vi "GeoData.vi"() -> ()   [LabVIEW 2017] (continued)
41013\tPost\tOR\tCrook County\tH1\n97756\t41013\tRedmond\tOR\tCrook County\tH1\n97406\t41015\tAgness\tOR\tCurry County\tH1\n97450\t41015\tLanglois\tOR\tCurry County\tH1\n97491\t41015\tWedderburn\tOR\tCurry County\tH1\n97444\t41015\tGold beach\tOR\tCurry County\tH1\n97476\t41015\tSixes\tOR\tCurry County\tH1\n97415\t41015\tBrookings\tOR\tCurry County\tH1\n97465\t41015\tPort orford\tOR\tCurry County\tH1\n97464\t41015\tOphir\tOR\tCurry County\tH1\n97709\t41017\tBend\tOR\tDeschutes County\tH1\n97701\t41017\tBend\tOR\tDeschutes County\tH1\n97759\t41017\tSisters\tOR\tDeschutes County\tH1\n97760\t41017\tTerrebonne\tOR\tDeschutes County\tH1\n97708\t41017\tBend\tOR\tDeschutes County\tH1\n97702\t41017\tBend\tOR\tDeschutes County\tH1\n97703\t41017\tBend\tOR\tDeschutes County\tH1\n97739\t41017\tLa pine\tOR\tDeschutes County\tH1\n97756\t41017\tRedmond\tOR\tDeschutes County\tH1\n97707\t41017\tBend\tOR\tDeschutes County\tH1\n97712\t41017\tBrothers\tOR\tDeschutes County\tH1\n97473\t41019\tScottsburg\tOR\tDouglas County\tH1\n97471\t41019\tRoseburg\tOR\tDouglas County\tH1\n97432\t41019\tDillard\tOR\tDouglas County\tH1\n97410\t41019\tAzalea\tOR\tDouglas County\tH1\n97443\t41019\tGlide\tOR\tDouglas County\tH1\n97481\t41019\tTenmile\tOR\tDouglas County\tH1\n97429\t41019\tDays creek\tOR\tDouglas County\tH1\n97442\t41019\tGlendale\tOR\tDouglas County\tH1\n97417\t41019\tCanyonville\tOR\tDouglas County\tH1\n97459\t41019\tNorth bend\tOR\tDouglas County\tH1\n97470\t41019\tRoseburg\tOR\tDouglas County\tH1\n97462\t41019\tOakland\tOR\tDouglas County\tH1\n97467\t41019\tReedsport\tOR\tDouglas County\tH1\n97469\t41019\tRiddle\tOR\tDouglas County\tH1\n97496\t41019\tWinston\tOR\tDouglas County\tH1\n97731\t41019\tChemult\tOR\tDouglas County\tH1\n97424\t41019\tCottage grove\tOR\tDouglas County\tH1\n97499\t41019\tYoncalla\tOR\tDouglas County\tH1\n97436\t41019\tElkton\tOR\tDouglas County\tH1\n97495\t41019\tWinchester\tOR\tDouglas County\tH1\n97486\t41019\tUmpqua\tOR\tDouglas County\tH1\n97441\t41019\tGardiner\tOR\tDouglas County\tH1\n97457\t41019\tMyrtle creek\tOR\tDouglas County\tH1\n97447\t41019\tIdleyld park\tOR\tDouglas County\tH1\n97435\t41019\tDrain\tOR\tDouglas County\tH1\n97493\t41019\tWestlake\tOR\tDouglas County\tH1\n97484\t41019\tTiller\tOR\tDouglas County\tH1\n97479\t41019\tSutherlin\tOR\tDouglas County\tH1\n97416\t41019\tCamas valley\tOR\tDouglas County\tH1\n97494\t41019\tWilbur\tOR\tDouglas County\tH1\n97843\t41021\tIone\tOR\tGilliam County\tH1\n97812\t41021\tArlington\tOR\tGilliam County\tH1\n97830\t41021\tFossil\tOR\tGilliam County\tH1\n97823\t41021\tCondon\tOR\tGilliam County\tH1\n97865\t41023\tMount vernon\tOR\tGrant County\tH1\n97856\t41023\tLong creek\tOR\tGrant County\tH1\n97820\t41023\tCanyon city\tOR\tGrant County\tH1\n97864\t41023\tMonument\tOR\tGrant County\tH1\n97817\t41023\tBates\tOR\tGrant County\tH1\n97825\t41023\tDayville\tOR\tGrant County\tH1\n97848\t41023\tKimberly\tOR\tGrant County\tH1\n97877\t41023\tSumpter\tOR\tGrant County\tH1\n97845\t41023\tJohn day\tOR\tGrant County\tH1\n97869\t41023\tPrairie city\tOR\tGrant County\tH1\n97873\t41023\tSeneca\tOR\tGrant County\tH1\n97710\t41025\tFields\tOR\tHarney County\tH1\n97721\t41025\tPrinceton\tOR\tHarney County\tH1\n97736\t41025\tFrenchglen\tOR\tHarney County\tH1\n97732\t41025\tCrane\tOR\tHarney County\tH1\n97758\t41025\tRiley\tOR\tHarney County\tH1\n97720\t41025\tBurns\tOR\tHarney County\tH1\n97904\t41025\tDrewsey\tOR\tHarney County\tH1\n97738\t41025\tHines\tOR\tHarney County\tH1\n97722\t41025\tDiamond\tOR\tHarney County\tH1\n97044\t41027\tOdell\tOR\tHood River County\tH1\n97014\t41027\tCascade locks\tOR\tHood River County\tH1\n97031\t41027\tHood river\tOR\tHood River County\tH1\n97041\t41027\tMount hood parkdale\tOR\tHood River County\tH1\n97526\t41029\tGrants pass\tOR\tJackson County\tH1\n97541\t41029\tTrail\tOR\tJackson County\tH1\n97502\t41029\tCentral point\tOR\tJackson County\tH1\n97524\t41029\tEagle point\tOR\tJackson County\tH1\n97527\t41029\tGrants pass\tOR\tJackson County\tH1\n97504\t41029\tMedford\tOR\tJackson County\tH1\n97530\t41029\tJacksonville\tOR\tJackson County\tH1\n97537\t41029\tRogue river\tOR\tJackson County\tH1\n97539\t41029\tShady cove\tOR\tJackson County\tH1\n97535\t41029\tPhoenix\tOR\tJackson County\tH1\n97520\t41029\tAshland\tOR\tJackson County\tH1\n97497\t41029\tWolf creek\tOR\tJackson County\tH1\n97540\t41029\tTalent\tOR\tJackson County\tH1\n97544\t41029\tWilliams\tOR\tJackson County\tH1\n97501\t41029\tMedford\tOR\tJackson County\tH1\n97503\t41029\tWhite city\tOR\tJackson County\tH1\n97525\t41029\tGold hill\tOR\tJackson County\tH1\n97522\t41029\tButte falls\tOR\tJackson County\tH1\n97536\t41029\tProspect\tOR\tJackson County\tH1\n97761\t41031\tWarm springs\tOR\tJefferson County\tH1\n97759\t41031\tSisters\tOR\tJefferson County\tH1\n97741\t41031\tMadras\tOR\tJefferson County\tH1\n97760\t41031\tTerrebonne\tOR\tJefferson County\tH1\n97711\t41031\tAshwood\tOR\tJefferson County\tH1\n97734\t41031\tCulver\tOR\tJefferson County\tH1\n97730\t41031\tCamp sherman\tOR\tJefferson County\tH1\n97526\t41033\tGrants pass\tOR\tJosephine County\tH1\n97531\t41033\tKerby\tOR\tJosephine County\tH1\n97527\t41033\tGrants pass\tOR\tJosephine County\tH1\n97543\t41033\tWilderville\tOR\tJosephine County\tH1\n97528\t41033\tGrants pass\tOR\tJosephine County\tH1\n97530\t41033\tJacksonville\tOR\tJosephine County\tH1\n97523\t41033\tCave junction\tOR\tJosephine County\tH1\n97532\t41033\tMerlin\tOR\tJosephine County\tH1\n97497\t41033\tWolf creek\tOR\tJosephine County\tH1\n97534\t41033\tO brien\tOR\tJosephine County\tH1\n97533\t41033\tMurphy\tOR\tJosephine County\tH1\n97544\t41033\tWilliams\tOR\tJosephine County\tH1\n97538\t41033\tSelma\tOR\tJosephine County\tH1\n97603\t41035\tKlamath falls\tOR\tKlamath County\tH1\n97601\t41035\tKlamath falls\tOR\tKlamath County\tH1\n97623\t41035\tBonanza\tOR\tKlamath County\tH1\n97627\t41035\tKeno\tOR\tKlamath County\tH1\n97621\t41035\tBeatty\tOR\tKlamath County\tH1\n97602\t41035\tKlamath falls\tOR\tKlamath County\tH1\n97604\t41035\tCrater lake\tOR\tKlamath County\tH1\n97625\t41035\tDairy\tOR\tKlamath County\tH1\n97731\t41035\tChemult\tOR\tKlamath County\tH1\n97739\t41035\tLa pine\tOR\tKlamath County\tH1\n97634\t41035\tMidland\tOR\tKlamath County\tH1\n97622\t41035\tBly\tOR\tKlamath County\tH1\n97624\t41035\tChiloquin\tOR\tKlamath County\tH1\n97733\t41035\tCrescent\tOR\tKlamath County\tH1\n97632\t41035\tMalin\tOR\tKlamath County\tH1\n97639\t41035\tSprague river\tOR\tKlamath County\tH1\n97626\t41035\tFort klamath\tOR\tKlamath County\tH1\n97633\t41035\tMerrill\tOR\tKlamath County\tH1\n97737\t41035\tGilchrist\tOR\tKlamath County\tH1\n97640\t41037\tSummer lake\tOR\tLake County\tH1\n97637\t41037\tPlush\tOR\tLake County\tH1\n97630\t41037\tLakeview\tOR\tLake County\tH1\n97641\t41037\tChristmas valley\tOR\tLake County\tH1\n97620\t41037\tAdel\tOR\tLake County\tH1\n97635\t41037\tNew pine creek\tOR\tLake County\tH1\n97638\t41037\tSilver lake\tOR\tLake County\tH1\n97735\t41037\tFort rock\tOR\tLake County\tH1\n97636\t41037\tPaisley\tOR\tLake County\tH1\n97413\t41039\tBlue river\tOR\tLane County\tH1\n97412\t41039\tBlachly\tOR\tLane County\tH1\n97402\t41039\tEugene\tOR\tLane County\tH1\n97404\t41039\tEugene\tOR\tLane County\tH1\n97454\t41039\tMarcola\tOR\tLane County\tH1\n97426\t41039\tCreswell\tOR\tLane County\tH1\n97487\t41039\tVeneta\tOR\tLane County\tH1\n97451\t41039\tLorane\tOR\tLane County\tH1\n97498\t41039\tYachats\tOR\tLane County\tH1\n97488\t41039\tVida\tOR\tLane County\tH1\n97461\t41039\tNoti\tOR\tLane County\tH1\n97324\t41039\tAlsea\tOR\tLane County\tH1\n97401\t41039\tEugene\tOR\tLane County\tH1\n97477\t41039\tSpringfield\tOR\tLane County\tH1\n97478\t41039\tSpringfield\tOR\tLane County\tH1\n97434\t41039\tDorena\tOR\tLane County\tH1\n97446\t41039\tHarrisburg\tOR\tLane County\tH1\n97463\t41039\tOakridge\tOR\tLane County\tH1\n97492\t41039\tWestfir\tOR\tLane County\tH1\n97409\t41039\tAlvadore\tOR\tLane County\tH1\n97438\t41039\tFall creek\tOR\tLane County\tH1\n97390\t41039\tTidewater\tOR\tLane County\tH1\n97490\t41039\tWalton\tOR\tLane County\tH1\n97489\t41039\tWalterville\tOR\tLane County\tH1\n97448\t41039\tJunction city\tOR\tLane County\tH1\n97453\t41039\tMapleton\tOR\tLane County\tH1\n97456\t41039\tMonroe\tOR\tLane County\tH1\n97480\t41039\tSwisshome\tOR\tLane County\tH1\n97405\t41039\tEugene\tOR\tLane County\tH1\n97424\t41039\tCottage grove\tOR\tLane County\tH1\n97439\t41039\tFlorence\tOR\tLane County\tH1\n97419\t41039\tCheshire\tOR\tLane County\tH1\n97437\t41039\tElmira\tOR\tLane County\tH1\n97452\t41039\tLowell\tOR\tLane County\tH1\n97430\t41039\tDeadwood\tOR\tLane County\tH1\n97408\t41039\tEugene\tOR\tLane County\tH1\n97493\t41039\tWestlake\tOR\tLane County\tH1\n97403\t41039\tEugene\tOR\tLane County\tH1\n97440\t41039\tEugene\tOR\tLane County\tH1\n97455\t41039\tPleasant hill\tOR\tLane County\tH1\n97475\t41039\tSpringfield\tOR\tLane County\tH1\n97431\t41039\tDexter\tOR\tLane County\tH1\n97394\t41041\tWaldport\tOR\tLincoln County\tH1\n97498\t41041\tYachats\tOR\tLincoln County\tH1\n97369\t41041\tOtter rock\tOR\tLincoln County\tH1\n97324\t41041\tAlsea\tOR\tLincoln County\tH1\n97391\t41041\tToledo\tOR\tLincoln County\tH1\n97364\t41041\tNeotsu\tOR\tLincoln County\tH1\n97367\t41041\tLincoln city\tOR\tLincoln County\tH1\n97390\t41041\tTidewater\tOR\tLincoln County\tH1\n97341\t41041\tDepoe bay\tOR\tLincoln County\tH1\n97380\t41041\tSiletz\tOR\tLincoln County\tH1\n97343\t41041\tEddyville\tOR\tLincoln County\tH1\n97388\t41041\tGleneden beach\tOR\tLincoln County\tH1\n97357\t41041\tLogsden\tOR\tLincoln County\tH1\n97376\t41041\tSeal rock\tOR\tLincoln County\tH1\n97365\t41041\tNewport\tOR\tLincoln County\tH1\n97368\t41041\tOtis\tOR\tLincoln County\tH1\n97366\t41041\tSouth beach\tOR\tLincoln County\tH1\n97326\t41041\tBlodgett\tOR\tLincoln County\tH1\n97346\t41043\tGates\tOR\tLinn County\tH1\n97333\t41043\tCorvallis\tOR\tLinn County\tH1\n97374\t41043\tScio\tOR\tLinn County\tH1\n97446\t41043\tHarrisburg\tOR\tLinn County\tH1\n97336\t41043\tCrawfordsville\tOR\tLinn County\tH1\n97355\t41043\tLebanon\tOR\tLinn County\tH1\n97383\t41043\tStayton\tOR\tLinn County\tH1\n97386\t41043\tSweet home\tOR\tLinn County\tH1\n97360\t41043\tMill city\tOR\tLinn County\tH1\n97350\t41043\tIdanha\tOR\tLinn County\tH1\n97327\t41043\tBrownsville\tOR\tLinn County\tH1\n97389\t41043\tTangent\tOR\tLinn County\tH1\n97377\t41043\tShedd\tOR\tLinn County\tH1\n97329\t41043\tCascadia\tOR\tLinn County\tH1\n97348\t41043\tHalsey\tOR\tLinn County\tH1\n97335\t41043\tCrabtree\tOR\tLinn County\tH1\n97358\t41043\tLyons\tOR\tLinn County\tH1\n97345\t41043\tFoster\tOR\tLinn County\tH1\n97322\t41043\tAlbany\tOR\tLinn County\tH1\n97321\t41043\tAlbany\tOR\tLinn County\tH1\n97352\t41043\tJefferson\tOR\tLinn County\tH1\n97906\t41045\tHarper\tOR\tMalheur County\tH1\n97908\t41045\tIronside\tOR\tMalheur County\tH1\n97910\t41045\tJordan valley\tOR\tMalheur County\tH1\n97920\t41045\tWestfall\tOR\tMalheur County\tH1\n97903\t41045\tBrogan\tOR\tMalheur County\tH1\n97918\t41045\tVale\tOR\tMalheur County\tH1\n97911\t41045\tJuntura\tOR\tMalheur County\tH1\n97913\t41045\tNyssa\tOR\tMalheur County\tH1\n97917\t41045\tRiverside\tOR\tMalheur County\tH1\n97902\t41045\tArock\tOR\tMalheur County\tH1\n97901\t41045\tAdrian\tOR\tMalheur County\tH1\n97909\t41045\tJamieson\tOR\tMalheur County\tH1\n97914\t41045\tOntario\tOR\tMalheur County\tH1\n97907\t41045\tHuntington\tOR\tMalheur County\tH1\n97137\t41047\tSaint paul\tOR\tMarion County\tH1\n97301\t41047\tSalem\tOR\tMarion County\tH1\n97346\t41047\tGates\tOR\tMarion County\tH1\n97342\t41047\tDetroit\tOR\tMarion County\tH1\n97306\t41047\tSalem\tOR\tMarion County\tH1\n97362\t41047\tMount angel\tOR\tMarion County\tH1\n97026\t41047\tGervais\tOR\tMarion County\tH1\n97308\t41047\tSalem\tOR\tMarion County\tH1\n97310\t41047\tSalem\tOR\tMarion County\tH1\n97373\t41047\tSaint benedict\tOR\tMarion County\tH1\n97317\t41047\tSalem\tOR\tMarion County\tH1\n97381\t41047\tSilverton\tOR\tMarion County\tH1\n97385\t41047\tSublimity\tOR\tMarion County\tH1\n97375\t41047\tScotts mills\tOR\tMarion County\tH1\n97071\t41047\tWoodburn\tOR\tMarion County\tH1\n97307\t41047\tKeizer\tOR\tMarion County\tH1\n97392\t41047\tTurner\tOR\tMarion County\tH1\n97383\t41047\tStayton\tOR\tMarion County\tH1\n97384\t41047\tMehama\tOR\tMarion County\tH1\n97360\t41047\tMill city\tOR\tMarion County\tH1\n97350\t41047\tIdanha\tOR\tMarion County\tH1\n97314\t41047\tSalem\tOR\tMarion County\tH1\n97358\t41047\tLyons\tOR\tMarion County\tH1\n97311\t41047\tSalem\tOR\tMarion County\tH1\n97312\t41047\tSalem\tOR\tMarion County\tH1\n97002\t41047\tAurora\tOR\tMarion County\tH1\n97302\t41047\tSalem\tOR\tMarion County\tH1\n97303\t41047\tSalem\tOR\tMarion County\tH1\n97020\t41047\tDonald\tOR\tMarion County\tH1\n97309\t41047\tSalem\tOR\tMarion County\tH1\n97325\t41047\tAumsville\tOR\tMarion County\tH1\n97305\t41047\tSalem\tOR\tMarion County\tH1\n97032\t41047\tHubbard\tOR\tMarion County\tH1\n97352\t41047\tJefferson\tOR\tMarion County\tH1\n97313\t41047\tSalem\tOR\tMarion County\tH1\n97843\t41049\tIone\tOR\tMorrow County\tH1\n97839\t41049\tLexington\tOR\tMorrow County\tH1\n97826\t41049\tEcho\tOR\tMorrow County\tH1\n97818\t41049\tBoardman\tOR\tMorrow County\tH1\n97836\t41049\tHeppner\tOR\tMorrow County\tH1\n97823\t41049\tCondon\tOR\tMorrow County\tH1\n97844\t41049\tIrrigon\tOR\tMorrow County\tH1\n97838\t41049\tHermiston\tOR\tMorrow County\tH1\n97882\t41049\tUmatilla\tOR\tMorrow County\tH1\n97205\t41051\tPortland\tOR\tMultnomah County\tH1\n97209\t41051\tPortland\tOR\tMultnomah County\tH1\n97221\t41051\tPortland\tOR\tMultnomah County\tH1\n97215\t41051\tPortland\tOR\tMultnomah County\tH1\n97286\t41051\tPortland\tOR\tMultnomah County\tH1\n97292\t41051\tPortland\tOR\tMultnomah County\tH1\n97293\t41051\tPortland\tOR\tMultnomah County\tH1\n97283\t41051\tPortland\tOR\tMultnomah County\tH1\n97253\t41051\tPortland\tOR\tMultnomah County\tH1\n97133\t41051\tNorth plains\tOR\tMultnomah County\tH1\n97220\t41051\tPortland\tOR\tMultnomah County\tH1\n97216\t41051\tPortland\tOR\tMultnomah County\tH1\n97217\t41051\tPortland\tOR\tMultnomah County\tH1\n97009\t41051\tBoring\tOR\tMultnomah County\tH1\n97208\t41051\tPortland\tOR\tMultnomah County\tH1\n97254\t41051\tPortland\tOR\tMultnomah County\tH1\n97206\t41051\tPortland\tOR\tMultnomah County\tH1\n97233\t41051\tPortland\tOR\tMultnomah County\tH1\n97296\t41051\tPortland\tOR\tMultnomah County\tH1\n97207\t41051\tPortland\tOR\tMultnomah County\tH1\n97203\t41051\tPortland\tOR\tMultnomah County\tH1\n97210\t41051\tPortland\tOR\tMultnomah County\tH1\n97236\t41051\tPortland\tOR\tMultnomah County\tH1\n97266\t41051\tPortland\tOR\tMultnomah County\tH1\n97204\t41051\tPortland\tOR\tMultnomah County\tH1\n97223\t41051\tPortland\tOR\tMultnomah County\tH1\n97225\t41051\tPortland\tOR\tMultnomah County\tH1\n97227\t41051\tPortland\tOR\tMultnomah County\tH1\n97218\t41051\tPortland\tOR\tMultnomah County\tH1\n97231\t41051\tPortland\tOR\tMultnomah County\tH1\n97030\t41051\tGresham\tOR\tMultnomah County\tH1\n97014\t41051\tCascade locks\tOR\tMultnomah County\tH1\n97060\t41051\tTroutdale\tOR\tMultnomah County\tH1\n97019\t41051\tCorbett\tOR\tMultnomah County\tH1\n97294\t41051\tPortland\tOR\tMultnomah County\tH1\n97238\t41051\tPortland\tOR\tMultnomah County\tH1\n97280\t41051\tPortland\tOR\tMultnomah County\tH1\n97290\t41051\tPortland\tOR\tMultnomah County\tH1\n97242\t41051\tPortland\tOR\tMultnomah County\tH1\n97282\t41051\tPortland\tOR\tMultnomah County\tH1\n97250\t41051\tPortland\tOR\tMultnomah County\tH1\n97214\t41051\tPortland\tOR\tMultnomah County\tH1\n97219\t41051\tPortland\tOR\tMultnomah County\tH1\n97024\t41051\tFairview\tOR\tMultnomah County\tH1\n97056\t41051\tScappoose\tOR\tMultnomah County\tH1\n97251\t41051\tPortland\tOR\tMultnomah County\tH1\n97201\t41051\tPortland\tOR\tMultnomah County\tH1\n97124\t41051\tHillsboro\tOR\tMultnomah County\tH1\n97211\t41051\tPortland\tOR\tMultnomah County\tH1\n97212\t41051\tPortland\tOR\tMultnomah County\tH1\n97222\t41051\tPortland\tOR\tMultnomah County\tH1\n97229\t41051\tPortland\tOR\tMultnomah County\tH1\n97239\t41051\tPortland\tOR\tMultnomah County\tH1\n97080\t41051\tGresham\tOR\tMultnomah County\tH1\n97202\t41051\tPortland\tOR\tMultnomah County\tH1\n97213\t41051\tPortland\tOR\tMultnomah County\tH1\n97230\t41051\tPortland\tOR\tMultnomah County\tH1\n97232\t41051\tPortland\tOR\tMultnomah County\tH1\n97035\t41051\tLake oswego\tOR\tMultnomah County\tH1\n97034\t41051\tLake oswego\tOR\tMultnomah County\tH1\n97252\t41051\tPortland\tOR\tMultnomah County\tH1\n97258\t41051\tPortland\tOR\tMultnomah County\tH1\n97240\t41051\tPortland\tOR\tMultnomah County\tH1\n97228\t41051\tPortland\tOR\tMultnomah County\tH1\n97010\t41051\tBridal veil\tOR\tMultnomah County\tH1\n97338\t41053\tDallas\tOR\tPolk County\tH1\n97344\t41053\tFalls city\tOR\tPolk County\tH1\n97371\t41053\tRickreall\tOR\tPolk County\tH1\n97351\t41053\tIndependence\tOR\tPolk County\tH1\n97347\t41053\tGrand ronde\tOR\tPolk County\tH1\n97396\t41053\tWillamina\tOR\tPolk County\tH1\n97378\t41053\tSheridan\tOR\tPolk County\tH1\n97101\t41053\tAmity\tOR\tPolk County\tH1\n97304\t41053\tSalem\tOR\tPolk County\tH1\n97361\t41053\tMonmouth\tOR\tPolk County\tH1\n97370\t41053\tPhilomath\tOR\tPolk County\tH1\n97039\t41055\tMoro\tOR\tSherman County\tH1\n97029\t41055\tGrass valley\tOR\tSherman County\tH1\n97050\t41055\tRufus\tOR\tSherman County\tH1\n97065\t41055\tWasco\tOR\tSherman County\tH1\n97033\t41055\tKent\tOR\tSherman County\tH1\n97112\t41057\tCloverdale\tOR\tTillamook County\tH1\n97149\t41057\tNeskowin\tOR\tTillamook County\tH1\n97102\t41057\tArch cape\tOR\tTillamook County\tH1\n97143\t41057\tNetarts\tOR\tTillamook County\tH1\n97147\t41057\tWheeler\tOR\tTillamook County\tH1\n97136\t41057\tRockaway beach\tOR\tTillamook County\tH1\n97107\t41057\tBay city\tOR\tTillamook County\tH1\n97141\t41057\tTillamook\tOR\tTillamook County\tH1\n97135\t41057\tPacific city\tOR\tTillamook County\tH1\n97134\t41057\tOceanside\tOR\tTillamook County\tH1\n97131\t41057\tNehalem\tOR\tTillamook County\tH1\n97118\t41057\tGaribaldi\tOR\tTillamook County\tH1\n97108\t41057\tBeaver\tOR\tTillamook County\tH1\n97130\t41057\tManzanita\tOR\tTillamook County\tH1\n97368\t41057\tOtis\tOR\tTillamook County\tH1\n97122\t41057\tHebo\tOR\tTillamook County\tH1\n97875\t41059\tStanfield\tOR\tUmatilla County\tH1\n97835\t41059\tHelix\tOR\tUmatilla County\tH1\n97826\t41059\tEcho\tOR\tUmatilla County\tH1\n97880\t41059\tUkiah\tOR\tUmatilla County\tH1\n97886\t41059\tWeston\tOR\tUmatilla County\tH1\n97801\t41059\tPendleton\tOR\tUmatilla County\tH1\n97813\t41059\tAthena\tOR\tUmatilla County\tH1\n97862\t41059\tMilton freewater\tOR\tUmatilla County\tH1\n97868\t41059\tPilot rock\tOR\tUmatilla County\tH1\n97859\t41059\tMeacham\tOR\tUmatilla County\tH1\n97838\t41059\tHermiston\tOR\tUmatilla County\tH1\n97810\t41059\tAdams\tOR\tUmatilla County\tH1\n97882\t41059\tUmatilla\tOR\tUmatilla County\tH1\n97883\t41061\tUnion\tOR\tUnion County\tH1\n97814\t41061\tBaker city\tOR\tUnion County\tH1\n97850\t41061\tLa grande\tOR\tUnion County\tH1\n97824\t41061\tCove\tOR\tUnion County\tH1\n97886\t41061\tWeston\tOR\tUnion County\tH1\n97867\t41061\tNorth powder\tOR\tUnion County\tH1\n97841\t41061\tImbler\tOR\tUnion County\tH1\n97827\t41061\tElgin\tOR\tUnion County\tH1\n97876\t41061\tSummerville\tOR\tUnion County\tH1\n97857\t41063\tLostine\tOR\tWallowa County\tH1\n97846\t41063\tJoseph\tOR\tWallowa County\tH1\n97842\t41063\tImnaha\tOR\tWallowa County\tH1\n97885\t41063\tWallowa\tOR\tWallowa County\tH1\n97828\t41063\tEnterprise\tOR\tWallowa County\tH1\n97827\t41063\tElgin\tOR\tWallowa County\tH1\n97021\t41065\tDufur\tOR\tWasco County\tH1\n97063\t41065\tTygh valley\tOR\tWasco County\tH1\n97037\t41065\tMaupin\tOR\tWasco County\tH1\n97058\t41065\tThe dalles\tOR\tWasco County\tH1\n97040\t41065\tMosier\tOR\tWasco County\tH1\n97001\t41065\tAntelope\tOR\tWasco County\tH1\n97057\t41065\tShaniko\tOR\tWasco County\tH1\n97005\t41067\tBeaverton\tOR\tWashington County\tH1\n97140\t41067\tSherwood\tOR\tWashington County\tH1\n97221\t41067\tPortland\tOR\tWashington County\tH1\n97007\t41067\tBeaverton\tOR\tWashington County\tH1\n97113\t41067\tCornelius\tOR\tWashington County\tH1\n97133\t41067\tNorth plains\tOR\tWashington County\tH1\n97129\t41067\tHillsboro\tOR\tWashington County\tH1\n97123\t41067\tHillsboro\tOR\tWashington County\tH1\n97062\t41067\tTualatin\tOR\tWashington County\tH1\n97119\t41067\tGaston\tOR\tWashington County\tH1\n97210\t41067\tPortland\tOR\tWashington County\tH1\n97078\t41067\tBeaverton\tOR\tWashington County\tH1\n97125\t41067\tManning\tOR\tWashington County\tH1\n97291\t41067\tPortland\tOR\tWashington County\tH1\n97079\t41067\tBeaverton\tOR\tWashington County\tH1\n97003\t41067\tBeaverton\tOR\tWashington County\tH1\n97223\t41067\tPortland\tOR\tWashington County\tH1\n97225\t41067\tPortland\tOR\tWashington County\tH1\n97231\t41067\tPortland\tOR\tWashington County\tH1\n97144\t41067\tTimber\tOR\tWashington County\tH1\n97298\t41067\tPortland\tOR\tWashington County\tH1\n97132\t41067\tNewberg\tOR\tWashington County\tH1\n97117\t41067\tGales creek\tOR\tWashington County\tH1\n97219\t41067\tPortland\tOR\tWashington County\tH1\n97056\t41067\tScappoose\tOR\tWashington County\tH1\n97006\t41067\tBeaverton\tOR\tWashington County\tH1\n97116\t41067\tForest grove\tOR\tWashington County\tH1\n97124\t41067\tHillsboro\tOR\tWashington County\tH1\n97106\t41067\tBanks\tOR\tWashington County\tH1\n97229\t41067\tPortland\tOR\tWashington County\tH1\n97224\t41067\tPortland\tOR\tWashington County\tH1\n97008\t41067\tBeaverton\tOR\tWashington County\tH1\n97109\t41067\tBuxton\tOR\tWashington County\tH1\n97281\t41067\tPortland\tOR\tWashington County\tH1\n97064\t41067\tVernonia\tOR\tWashington County\tH1\n97035\t41067\tLake oswego\tOR\tWashington County\tH1\n97070\t41067\tWilsonville\tOR\tWashington County\tH1\n97075\t41067\tBeaverton\tOR\tWashington County\tH1\n97750\t41069\tMitchell\tOR\tWheeler County\tH1\n97874\t41069\tSpray\tOR\tWheeler County\tH1\n97830\t41069\tFossil\tOR\tWheeler County\tH1\n97823\t41069\tCondon\tOR\tWheeler County\tH1\n97114\t41071\tDayton\tOR\tYamhill County\tH1\n97140\t41071\tSherwood\tOR\tYamhill County\tH1\n97115\t41071\tDundee\tOR\tYamhill County\tH1\n97347\t41071\tGrand ronde\tOR\tYamhill County\tH1\n97396\t41071\tWillamina\tOR\tYamhill County\tH1\n97123\t41071\tHillsboro\tOR\tYamhill County\tH1\n97128\t41071\tMcminnville\tOR\tYamhill County\tH1\n97111\t41071\tCarlton\tOR\tYamhill County\tH1\n97119\t41071\tGaston\tOR\tYamhill County\tH1\n97132\t41071\tNewberg\tOR\tYamhill County\tH1\n97127\t41071\tLafayette\tOR\tYamhill County\tH1\n97378\t41071\tSheridan\tOR\tYamhill County\tH1\n97101\t41071\tAmity\tOR\tYamhill County\tH1\n97304\t41071\tSalem\tOR\tYamhill County\tH1\n97148\t41071\tYamhill\tOR\tYamhill County\tH1\n17320\t42001\tFairfield\tPA\tAdams County\tH1\n17340\t42001\tLittlestown\tPA\tAdams County\tH1\n17306\t42001\tBendersville\tPA\tAdams County\tH1\n17222\t42001\tFayetteville\tPA\tAdams County\tH1\n17307\t42001\tBiglerville\tPA\tAdams County\tH1\n17301\t42001\tAbbottstown\tPA\tAdams County\tH1\n17325\t42001\tGettysburg\tPA\tAdams County\tH1\n17331\t42001\tHanover\tPA\tAdams County\tH1\n17324\t42001\tGardners\tPA\tAdams County\tH1\n17316\t42001\tEast berlin\tPA\tAdams County\tH1\n17337\t42001\tIdaville\tPA\tAdams County\tH1\n17310\t42001\tCashtown\tPA\tAdams County\tH1\n17019\t42001\tDillsburg\tPA\tAdams County\tH1\n17344\t42001\tMc sherrystown\tPA\tAdams County\tH1\n17375\t42001\tPeach glen\tPA\tAdams County\tH1\n17343\t42001\tMc knightstown\tPA\tAdams County\tH1\n17304\t42001\tAspers\tPA\tAdams County\tH1\n17350\t42001\tNew oxford\tPA\tAdams County\tH1\n17372\t42001\tYork springs\tPA\tAdams County\tH1\n17353\t42001\tOrrtanna\tPA\tAdams County\tH1\n17303\t42001\tArendtsville\tPA\tAdams County\tH1\n15034\t42003\tDravosburg\tPA\tAllegheny County\tH1\n15135\t42003\tMckeesport\tPA\tAllegheny County\tH1\n15218\t42003\tPittsburgh\tPA\tAllegheny County\tH1\n15230\t42003\tPittsburgh\tPA\tAllegheny County\tH1\n15227\t42003\tPittsburgh\tPA\tAllegheny County\tH1\n15046\t42003\tCrescent\tPA\tAllegheny County\tH1\n15215\t42003\tPittsburgh\tPA\tAllegheny County\tH1\n15088\t42003\tWest elizabeth\tPA\tAllegheny County\tH1\n15259\t42003\tPittsburgh\tPA\tAllegheny County\tH1\n15001\t42003\tAliquippa\tPA\tAllegheny County\tH1\n15012\t42003\tBelle vernon\tPA\tAllegheny County\tH1\n15024\t42003\tCheswick\tPA\tAllegheny County\tH1\n15035\t42003\tEast mc keesport\tPA\tAllegheny County\tH1\n15047\t42003\tGreenock\tPA\tAllegheny County\tH1\n15071\t42003\tOakdale\tPA\tAllegheny County\tH1\n15104\t42003\tBraddock\tPA\tAllegheny County\tH1\n15142\t42003\tPresto\tPA\tAllegheny County\tH1\n15122\t42003\tWest mifflin\tPA\tAllegheny County\tH1\n15139\t42003\tOakmont\tPA\tAllegheny County\tH1\n15137\t42003\tNorth versailles\tPA\tAllegheny County\tH1\n15144\t42003\tSpringdale\tPA\tAllegheny County\tH1\n15228\t42003\tPittsburgh\tPA\tAllegheny County\tH1\n15237\t42003\tPittsburgh\tPA\tAllegheny County\tH1\n15233\t42003\tPittsburgh\tPA\tAllegheny County\tH1\n15642\t42003\tIrwin\tPA\tAllegheny County\tH1\n16059\t42003\tValencia\tPA\tAllegheny County\tH1\n15014\t42003\tBrackenridge\tPA\tAllegheny County\tH1\n15321\t42003\tCecil\tPA\tAllegheny County\tH1\n15290\t42003\tPittsburgh\tPA\tAllegheny County\tH1\n15006\t42003\tBairdford\tPA\tAllegheny County\tH1\n15091\t42003\tWildwood\tPA\tAllegheny County\tH1\n15253\t42003\tPittsburgh\tPA\tAllegheny County\tH1\n15267\t42003\tPittsburgh\tPA\tAllegheny County\tH1\n15017\t42003\tBridgeville\tPA\tAllegheny County\tH1\n15044\t42003\tGibsonia\tPA\tAllegheny County\tH1\n15026\t42003\tClinton\tPA\tAllegheny County\tH1\n15116\t42003\tGlenshaw\tPA\tAllegheny County\tH1\n15202\t42003\tPittsburgh\tPA\tAllegheny County\tH1\n15209\t42003\tPittsburgh\tPA\tAllegheny County\tH1\n15216\t42003\tPittsburgh\tPA\tAllegheny County\tH1\n15221\t42003\tPittsburgh\tPA\tAllegheny County\tH1\n15236\t42003\tPittsburgh\tPA\tAllegheny County\tH1\n15275\t42003\tPittsburgh\tPA\tAllegheny County\tH1\n15239\t42003\tPittsburgh\tPA\tAllegheny County\tH1\n15243\t42003\tPittsburgh\tPA\tAllegheny County\tH1\n15007\t42003\tBakerstown\tPA\tAllegheny County\tH1\n15031\t42003\tCuddy\tPA\tAllegheny County\tH1\n15032\t42003\tCurtisville\tPA\tAllegheny County\tH1\n15258\t42003\tPittsburgh\tPA\tAllegheny County\tH1\n15005\t42003\tBaden\tPA\tAllegheny County\tH1\n15101\t42003\tAllison park\tPA\tAllegheny County\tH1\n15102\t42003\tBethel park\tPA\tAllegheny County\tH1\n15129\t42003\tSouth park\tPA\tAllegheny County\tH1\n15145\t42003\tTurtle creek\tPA\tAllegheny County\tH1\n15126\t42003\tImperial\tPA\tAllegheny County\tH1\n15206\t42003\tPittsburgh\tPA\tAllegheny County\tH1\n15210\t42003\tPittsburgh\tPA\tAllegheny County\tH1\n15207\t42003\tPittsburgh\tPA\tAllegheny County\tH1\n15148\t42003\tWilmerding\tPA\tAllegheny County\tH1\n15220\t42003\tPittsburgh\tPA\tAllegheny County\tH1\n15226\t42003\tPittsburgh\tPA\tAllegheny County\tH1\n15332\t42003\tFinleyville\tPA\tAllegheny County\tH1\n15261\t42003\tPittsburgh\tPA\tAllegheny County\tH1\n15260\t42003\tPittsburgh\tPA\tAllegheny County\tH1\n15051\t42003\tIndianola\tPA\tAllegheny County\tH1\n15231\t42003\tPittsburgh\tPA\tAllegheny County\tH1\n15127\t42003\tIngomar\tPA\tAllegheny County\tH1\n15064\t42003\tMorgan\tPA\tAllegheny County\tH1\n15289\t42003\tPittsburgh\tPA\tAllegheny County\tH1\n15096\t42003\tWarrendale\tPA\tAllegheny County\tH1\n15018\t42003\tBuena vista\tPA\tAllegheny County\tH1\n15037\t42003\tElizabeth\tPA\tAllegheny County\tH1\n15068\t42003\tNew kensington\tPA\tAllegheny County\tH1\n15045\t42003\tGlassport\tPA\tAllegheny County\tH1\n15090\t42003\tWexford\tPA\tAllegheny County\tH1\n15089\t42003\tWest newton\tPA\tAllegheny County\tH1\n15083\t42003\tSutersville\tPA\tAllegheny County\tH1\n15136\t42003\tMc kees rocks\tPA\tAllegheny County\tH1\n15204\t42003\tPittsburgh\tPA\tAllegheny County\tH1\n15205\t42003\tPittsburgh\tPA\tAllegheny County\tH1\n15208\t42003\tPittsburgh\tPA\tAllegheny County\tH1\n15212\t42003\tPittsburgh\tPA\tAllegheny County\tH1\n15222\t42003\tPittsburgh\tPA\tAllegheny County\tH1\n15234\t42003\tPittsburgh\tPA\tAllegheny County\tH1\n15317\t42003\tCanonsburg\tPA\tAllegheny County\tH1\n15056\t42003\tLeetsdale\tPA\tAllegheny County\tH1\n15086\t42003\tWarrendale\tPA\tAllegheny County\tH1\n15134\t42003\tMckeesport\tPA\tAllegheny County\tH1\n15277\t42003\tPittsburgh\tPA\tAllegheny County\tH1\n15262\t42003\tPittsburgh\tPA\tAllegheny County\tH1\n15025\t42003\tClairton\tPA\tAllegheny County\tH1\n15065\t42003\tNatrona heights\tPA\tAllegheny County\tH1\n15057\t42003\tMc donald\tPA\tAllegheny County\tH1\n15049\t42003\tHarwick\tPA\tAllegheny County\tH1\n15108\t42003\tCoraopolis\tPA\tAllegheny County\tH1\n15106\t42003\tCarnegie\tPA\tAllegheny County\tH1\n15112\t42003\tEast pittsburgh\tPA\tAllegheny County\tH1\n15146\t42003\tMonroeville\tPA\tAllegheny County\tH1\n15120\t42003\tHomestead\tPA\tAllegheny County\tH1\n15131\t42003\tMckeesport\tPA\tAllegheny County\tH1\n15147\t42003\tVerona\tPA\tAllegheny County\tH1\n15213\t42003\tPittsburgh\tPA\tAllegheny County\tH1\n15219\t42003\tPittsburgh\tPA\tAllegheny County\tH1\n15241\t42003\tPittsburgh\tPA\tAllegheny County\tH1\n15244\t42003\tPittsburgh\tPA\tAllegheny County\tH1\n15211\t42003\tPittsburgh\tPA\tAllegheny County\tH1\n15015\t42003\tBradfordwoods\tPA\tAllegheny County\tH1\n15282\t42003\tPittsburgh\tPA\tAllegheny County\tH1\n15020\t42003\tBunola\tPA\tAllegheny County\tH1\n15110\t42003\tDuquesne\tPA\tAllegheny County\tH1\n15132\t42003\tMckeesport\tPA\tAllegheny County\tH1\n15201\t42003\tPittsburgh\tPA\tAllegheny County\tH1\n15214\t42003\tPittsburgh\tPA\tAllegheny County\tH1\n15217\t42003\tPittsburgh\tPA\tAllegheny County\tH1\n15224\t42003\tPittsburgh\tPA\tAllegheny County\tH1\n15235\t42003\tPittsburgh\tPA\tAllegheny County\tH1\n15232\t42003\tPittsburgh\tPA\tAllegheny County\tH1\n15225\t42003\tPittsburgh\tPA\tAllegheny County\tH1\n16046\t42003\tMars\tPA\tAllegheny County\tH1\n15030\t42003\tCreighton\tPA\tAllegheny County\tH1\n15123\t42003\tWest mifflin\tPA\tAllegheny County\tH1\n15038\t42003\tElrama\tPA\tAllegheny County\tH1\n15265\t42003\tPittsburgh\tPA\tAllegheny County\tH1\n15075\t42003\tRural ridge\tPA\tAllegheny County\tH1\n15082\t42003\tSturgeon\tPA\tAllegheny County\tH1\n15003\t42003\tAmbridge\tPA\tAllegheny County\tH1\n15063\t42003\tMonongahela\tPA\tAllegheny County\tH1\n15084\t42003\tTarentum\tPA\tAllegheny County\tH1\n15085\t42003\tTrafford\tPA\tAllegheny County\tH1\n15133\t42003\tMckeesport\tPA\tAllegheny County\tH1\n15143\t42003\tSewickley\tPA\tAllegheny County\tH1\n15140\t42003\tPitcairn\tPA\tAllegheny County\tH1\n15203\t42003\tPittsburgh\tPA\tAllegheny County\tH1\n15238\t42003\tPittsburgh\tPA\tAllegheny County\tH1\n15223\t42003\tPittsburgh\tPA\tAllegheny County\tH1\n15229\t42003\tPittsburgh\tPA\tAllegheny County\tH1\n16055\t42003\tSarver\tPA\tAllegheny County\tH1\n16229\t42003\tFreeport\tPA\tAllegheny County\tH1\n15076\t42003\tRussellton\tPA\tAllegheny County\tH1\n15240\t42003\tPittsburgh\tPA\tAllegheny County\tH1\n15276\t42003\tPittsburgh\tPA\tAllegheny County\tH1\n15295\t42003\tPittsburgh\tPA\tAllegheny County\tH1\n15272\t42003\tPittsburgh\tPA\tAllegheny County\tH1\n15028\t42003\tCoulters\tPA\tAllegheny County\tH1\n15095\t42003\tWarrendale\tPA\tAllegheny County\tH1\n15690\t42005\tVandergrift\tPA\tArmstrong County\tH1\n16028\t42005\tEast brady\tPA\tArmstrong County\tH1\n16224\t42005\tFairmount city\tPA\tArmstrong County\tH1\n15686\t42005\tSpring church\tPA\tArmstrong County\tH1\n16212\t42005\tCadogan\tPA\tArmstrong County\tH1\n15656\t42005\tLeechburg\tPA\tArmstrong County\tH1\n15613\t42005\tApollo\tPA\tArmstrong County\tH1\n16210\t42005\tAdrian\tPA\tArmstrong County\tH1\n16242\t42005\tNew bethlehem\tPA\tArmstrong County\tH1\n16041\t42005\tKarns city\tPA\tArmstrong County\tH1\n16222\t42005\tDayton\tPA\tArmstrong County\tH1\n16228\t42005\tFord cliff\tPA\tArmstrong County\tH1\n16263\t42005\tYatesboro\tPA\tArmstrong County\tH1\n16245\t42005\tOak ridge\tPA\tArmstrong County\tH1\n15774\t42005\tShelocta\tPA\tArmstrong County\tH1\n16049\t42005\tParker\tPA\tArmstrong County\tH1\n16226\t42005\tFord city\tPA\tArmstrong County\tH1\n16236\t42005\tMc grann\tPA\tArmstrong County\tH1\n15618\t42005\tAvonmore\tPA\tArmstrong County\tH1\n16201\t42005\tKittanning\tPA\tArmstrong County\tH1\n15732\t42005\tCreekside\tPA\tArmstrong County\tH1\n16025\t42005\tChicora\tPA\tArmstrong County\tH1\n16262\t42005\tWorthington\tPA\tArmstrong County\tH1\n16253\t42005\tSeminole\tPA\tArmstrong County\tH1\n15673\t42005\tNorth apollo\tPA\tArmstrong County\tH1\n15736\t42005\tElderton\tPA\tArmstrong County\tH1\n16240\t42005\tMayport\tPA\tArmstrong County\tH1\n16023\t42005\tCabot\tPA\tArmstrong County\tH1\n16238\t42005\tManorville\tPA\tArmstrong County\tH1\n16261\t42005\tWidnoon\tPA\tArmstrong County\tH1\n15682\t42005\tSchenley\tPA\tArmstrong County\tH1\n15681\t42005\tSaltsburg\tPA\tArmstrong County\tH1\n16218\t42005\tCowansville\tPA\tArmstrong County\tH1\n16244\t42005\tNu mine\tPA\tArmstrong County\tH1\n16055\t42005\tSarver\tPA\tArmstrong County\tH1\n16249\t42005\tRural valley\tPA\tArmstrong County\tH1\n16229\t42005\tFreeport\tPA\tArmstrong County\tH1\n16259\t42005\tTempleton\tPA\tArmstrong County\tH1\n16250\t42005\tSagamore\tPA\tArmstrong County\tH1\n15061\t42007\tMonaca\tPA\tBeaver County\tH1\n15019\t42007\tBulger\tPA\tBeaver County\tH1\n16136\t42007\tKoppel\tPA\tBeaver County\tH1\n15001\t42007\tAliquippa\tPA\tBeaver County\tH1\n15050\t42007\tHookstown\tPA\tBeaver County\tH1\n15066\t42007\tNew brighton\tPA\tBeaver County\tH1\n15059\t42007\tMidland\tPA\tBeaver County\tH1\n15074\t42007\tRochester\tPA\tBeaver County\tH1\n15081\t42007\tSouth heights\tPA\tBeaver County\tH1\n15026\t42007\tClinton\tPA\tBeaver County\tH1\n16120\t42007\tEnon valley\tPA\tBeaver County\tH1\n16063\t42007\tZelienople\tPA\tBeaver County\tH1\n16117\t42007\tEllwood city\tPA\tBeaver County\tH1\n15005\t42007\tBaden\tPA\tBeaver County\tH1\n15021\t42007\tBurgettstown\tPA\tBeaver County\tH1\n15126\t42007\tImperial\tPA\tBeaver County\tH1\n16123\t42007\tFombell\tPA\tBeaver County\tH1\n15077\t42007\tShippingport\tPA\tBeaver County\tH1\n15010\t42007\tBeaver falls\tPA\tBeaver County\tH1\n15009\t42007\tBeaver\tPA\tBeaver County\tH1\n15052\t42007\tIndustry\tPA\tBeaver County\tH1\n16157\t42007\tWampum\tPA\tBeaver County\tH1\n15042\t42007\tFreedom\tPA\tBeaver County\tH1\n16115\t42007\tDarlington\tPA\tBeaver County\tH1\n16141\t42007\tNew galilee\tPA\tBeaver County\tH1\n15003\t42007\tAmbridge\tPA\tBeaver County\tH1\n15027\t42007\tConway\tPA\tBeaver County\tH1\n15143\t42007\tSewickley\tPA\tBeaver County\tH1\n16037\t42007\tHarmony\tPA\tBeaver County\tH1\n15043\t42007\tGeorgetown\tPA\tBeaver County\tH1\n16655\t42009\tImler\tPA\tBedford County\tH1\n17211\t42009\tArtemas\tPA\tBedford County\tH1\n16670\t42009\tQueen\tPA\tBedford County\tH1\n15535\t42009\tClearville\tPA\tBedford County\tH1\n15550\t42009\tManns choice\tPA\tBedford County\tH1\n15946\t42009\tPortage\tPA\tBedford County\tH1\n16650\t42009\tHopewell\tPA\tBedford County\tH1\n16657\t42009\tJames creek\tPA\tBedford County\tH1\n15545\t42009\tHyndman\tPA\tBedford County\tH1\n15533\t42009\tBreezewood\tPA\tBedford County\tH1\n15926\t42009\tCentral city\tPA\tBedford County\tH1\n15522\t42009\tBedford\tPA\tBedford County\tH1\n16659\t42009\tLoysburg\tPA\tBedford County\tH1\n15539\t42009\tFishertown\tPA\tBedford County\tH1\n15554\t42009\tNew paris\tPA\tBedford County\tH1\n15521\t42009\tAlum bank\tPA\tBedford County\tH1\n16625\t42009\tClaysburg\tPA\tBedford County\tH1\n16695\t42009\tWoodbury\tPA\tBedford County\tH1\n16679\t42009\tSix mile run\tPA\tBedford County\tH1\n16667\t42009\tOsterburg\tPA\tBedford County\tH1\n16672\t42009\tRiddlesburg\tPA\tBedford County\tH1\n15537\t42009\tEverett\tPA\tBedford County\tH1\n15963\t42009\tWindber\tPA\tBedford County\tH1\n16678\t42009\tSaxton\tPA\tBedford County\tH1\n16633\t42009\tDefiance\tPA\tBedford County\tH1\n15530\t42009\tBerlin\tPA\tBedford County\tH1\n15559\t42009\tSchellsburg\tPA\tBedford County\tH1\n16664\t42009\tNew enterprise\tPA\tBedford County\tH1\n16673\t42009\tRoaring spring\tPA\tBedford County\tH1\n16662\t42009\tMartinsburg\tPA\tBedford County\tH1\n15534\t42009\tBuffalo mills\tPA\tBedford County\tH1\n18092\t42011\tZionsville\tPA\tBerks County\tH1\n19508\t42011\tBirdsboro\tPA\tBerks County\tH1\n19567\t42011\tWomelsdorf\tPA\tBerks County\tH1\n19554\t42011\tShartlesville\tPA\tBerks County\tH1\n19562\t42011\tTopton\tPA\tBerks County\tH1\n19533\t42011\tLeesport\tPA\tBerks County\tH1\n17087\t42011\tRichland\tPA\tBerks County\tH1\n19539\t42011\tMertztown\tPA\tBerks County\tH1\n19519\t42011\tEarlville\tPA\tBerks County\tH1\n19540\t42011\tMohnton\tPA\tBerks County\tH1\n19609\t42011\tReading\tPA\tBerks County\tH1\n19605\t42011\tReading\tPA\tBerks County\tH1\n19511\t42011\tBowers\tPA\tBerks County\tH1\n19550\t42011\tRehrersburg\tPA\tBerks County\tH1\n19523\t42011\tGeigertown\tPA\tBerks County\tH1\n17555\t42011\tNarvon\tPA\tBerks County\tH1\n18056\t42011\tHereford\tPA\tBerks County\tH1\n19505\t42011\tBechtelsville\tPA\tBerks County\tH1\n19512\t42011\tBoyertown\tPA\tBerks County\tH1\n19507\t42011\tBethel\tPA\tBerks County\tH1\n19530\t42011\tKutztown\tPA\tBerks County\tH1\n19541\t42011\tMohrsville\tPA\tBerks County\tH1\n19503\t42011\tBally\tPA\tBerks County\tH1\n19543\t42011\tMorgantown\tPA\tBerks County\tH1\n19612\t42011\tReading\tPA\tBerks County\tH1\n17026\t42011\tFredericksburg\tPA\tBerks County\tH1\n18041\t42011\tEast greenville\tPA\tBerks County\tH1\n19510\t42011\tBlandon\tPA\tBerks County\tH1\n19555\t42011\tShoemakersville\tPA\tBerks County\tH1\n19525\t42011\tGilbertsville\tPA\tBerks County\tH1\n19610\t42011\tReading\tPA\tBerks County\tH1\n19545\t42011\tNew berlinville\tPA\tBerks County\tH1\n19564\t42011\tVirginville\tPA\tBerks County\tH1\n18011\t42011\tAlburtis\tPA\tBerks County\tH1\n18062\t42011\tMacungie\tPA\tBerks County\tH1\n19506\t42011\tBernville\tPA\tBerks County\tH1\n19560\t42011\tTemple\tPA\tBerks County\tH1\n19526\t42011\tHamburg\tPA\tBerks County\tH1\n19520\t42011\tElverson\tPA\tBerks County\tH1\n19607\t42011\tReading\tPA\tBerks County\tH1\n19611\t42011\tReading\tPA\tBerks County\tH1\n19464\t42011\tPottstown\tPA\tBerks County\tH1\n17073\t42011\tNewmanstown\tPA\tBerks County\tH1\n19602\t42011\tReading\tPA\tBerks County\tH1\n19601\t42011\tReading\tPA\tBerks County\tH1\n19604\t42011\tReading\tPA\tBerks County\tH1\n19522\t42011\tFleetwood\tPA\tBerks County\tH1\n19551\t42011\tRobesonia\tPA\tBerks County\tH1\n19547\t42011\tOley\tPA\tBerks County\tH1\n19608\t42011\tReading\tPA\tBerks County\tH1\n19534\t42011\tLenhartsville\tPA\tBerks County\tH1\n19544\t42011\tMount aetna\tPA\tBerks County\tH1\n19538\t42011\tMaxatawny\tPA\tBerks County\tH1\n19548\t42011\tPine forge\tPA\tBerks County\tH1\n19535\t42011\tLimekiln\tPA\tBerks County\tH1\n18070\t42011\tPalm\tPA\tBerks County\tH1\n19518\t42011\tDouglassville\tPA\tBerks County\tH1\n19565\t42011\tWernersville\tPA\tBerks County\tH1\n19501\t42011\tAdamstown\tPA\tBerks County\tH1\n19536\t42011\tLyon station\tPA\tBerks County\tH1\n17067\t42011\tMyerstown\tPA\tBerks County\tH1\n17569\t42011\tReinholds\tPA\tBerks County\tH1\n18031\t42011\tBreinigsville\tPA\tBerks County\tH1\n19504\t42011\tBarto\tPA\tBerks County\tH1\n19603\t42011\tReading\tPA\tBerks County\tH1\n19529\t42011\tKempton\tPA\tBerks County\tH1\n19606\t42011\tReading\tPA\tBerks County\tH1\n19559\t42011\tStrausstown\tPA\tBerks County\tH1\n19516\t42011\tCenterport\tPA\tBerks County\tH1\n16637\t42013\tEast freedom\tPA\tBlair County\tH1\n16655\t42013\tImler\tPA\tBlair County\tH1\n15946\t42013\tPortage\tPA\tBlair County\tH1\n16601\t42013\tAltoona\tPA\tBlair County\tH1\n16611\t42013\tAlexandria\tPA\tBlair County\tH1\n16617\t42013\tBellwood\tPA\tBlair County\tH1\n16693\t42013\tWilliamsburg\tPA\tBlair County\tH1\n16603\t42013\tAltoona\tPA\tBlair County\tH1\n16684\t42013\tTipton\tPA\tBlair County\tH1\n16665\t42013\tNewry\tPA\tBlair County\tH1\n16636\t42013\tDysart\tPA\tBlair County\tH1\n16625\t42013\tClaysburg\tPA\tBlair County\tH1\n16648\t42013\tHollidaysburg\tPA\tBlair County\tH1\n16641\t42013\tGallitzin\tPA\tBlair County\t
